vi "Data Type to String.vi"(8 "error in (no error)":errorcluster, 11 "Data Type":refnum<class "Data Type.lvclass">) -> (0 "error out":errorcluster, 3 "String out":string)   [LabVIEW 2020, in "String.lvclass"]
uses:
  <vilib>/gpm_packages/@cs/data-type-serializer/source/String/String.lvclass
  <vilib>/gpm_packages/@cs/data-type-serializer/source/Data Type/Data Type.lvclass
  <vilib>/gpm_packages/@cs/data-type-serializer/source/String/String.lvclass/String.ctl
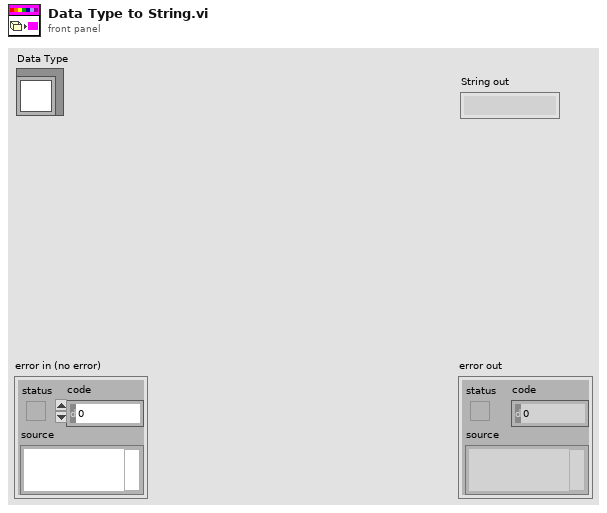
[diagram p1: front panel]
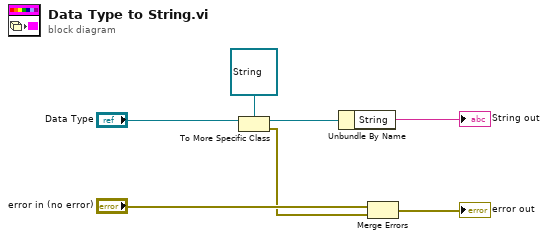
[diagram p0: block diagram]
diagram:
  n1 = To More Specific Class(target class=refnum<class "String.lvclass"> refnum ("Boolean out"), reference="Data Type") -> (specific class reference=w4:refnum<class "String.lvclass">, error out=w1:errorcluster)  [unwired: 1 in]
  n2 = Unbundle By Name(w4) -> ("String"=→"String out":string)
  n3 = Merge Errors("error in (no error)", w1) -> (→"error out":errorcluster)
